vi "TestGUI.vi"() -> ()   [LabVIEW 2020, in "VolatusScratch.lvlib"]
uses:
  VolatusScratch.lvlib
panel:
  out "DblControl":T1
  out "E":cluster{"Color":u32, "Value":dbl}
  out "D":dbl
  out "C":dbl
  out "B":dbl
  out "A":dbl
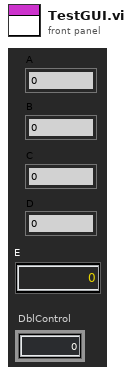
[diagram p1: front panel]
types:
  T1 = cluster{"Color":u32, "Value":dbl, "Backdrop":bool}
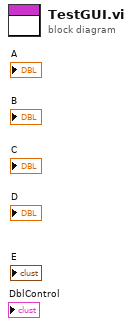
[diagram p0: block diagram]
diagram:
